vi "Smart Dashboard.vi"() -> ()   [LabVIEW 2017]
panel:
  in  "Smart Dashboard":enum32{"Smart Dashboard", "Tree", "Live Values"}(tab)
  out "Close":bool
  out "Open":bool
  out "String Array":string[](array[string])
  out "Boolean Array":bool[](array[boolean])
  out "Numeric Array":dbl[](array[numeric])
  out "String":string
  out "Boolean":bool
  out "Numeric":dbl
  in  "String Array":string[](array[string])
  in  "Boolean Array":bool[](array[boolean])
  in  "Numeric Array":dbl[](array[numeric])
  in  "String":string
  in  "Boolean":bool
  in  "Numeric":dbl
  out "Tree":string(tree)
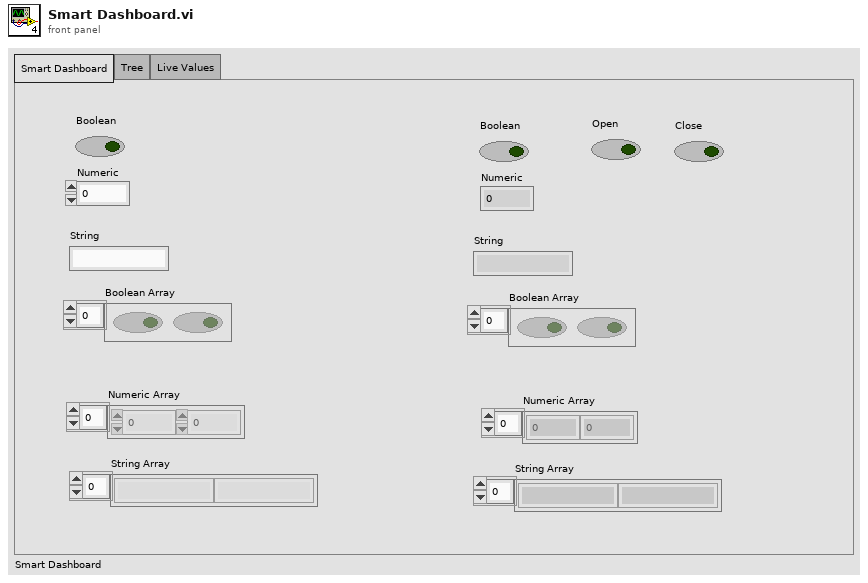
[diagram p1: front panel]
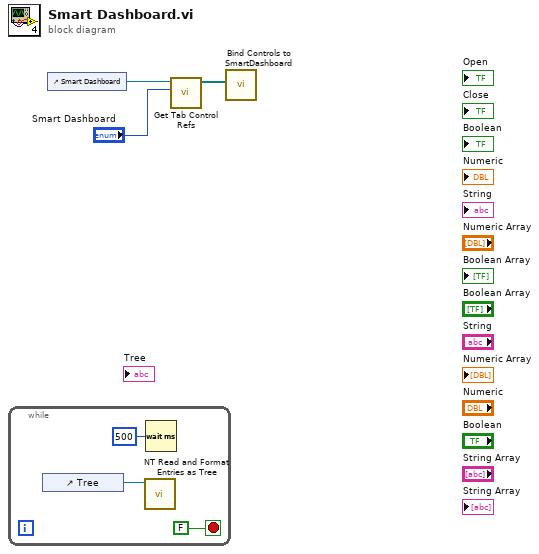
[diagram p0: block diagram]
diagram:
  n1 = while {
    stop <- FALSE stop-if-true
    n2 = control-ref of="Tree"() -> (w6:refnum<vi>)
    n3 = call <vilib>:"NT Read and Format Entries as Tree.vi"("Tree Refnum"=w6) -> ()  [unwired: 9 in, 2 out]
    n4 = Wait (ms)(milliseconds to wait=u32 500) -> ()  [unwired: 1 out]
  }
  n5 = control-ref of="Smart Dashboard"() -> (w3:refnum<vi>)
  n6 = call <vilib>:"Get Tab Control Refs.vi"("Page Index"="Smart Dashboard", "TabControl in"=w3) -> ("ControlsOnPage"=w1:refnum<vi>[])  [unwired: 9 in]
  n7 = call <vilib>:"Bind Controls to SmartDashboard.vi"("Bound Control Refs"=w1) -> ()  [unwired: 11 in]
